vi "Siargo Serial Number.vi"(8 "error in (no error)":errorcluster, 11 "Modbus API in":refnum<class "Modbus API.lvclass">) -> (0 "error out":errorcluster, 2 "Serial Number":string="*G7AEI02058*", 3 "Modbus API out":refnum<class "Modbus API.lvclass">)   [LabVIEW 2020]
uses:
  <vilib>/NI/Modbus Library/API/Modbus API.lvclass
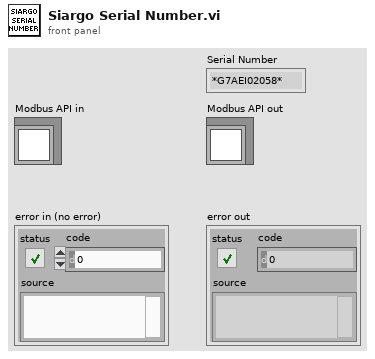
[diagram p1: front panel]
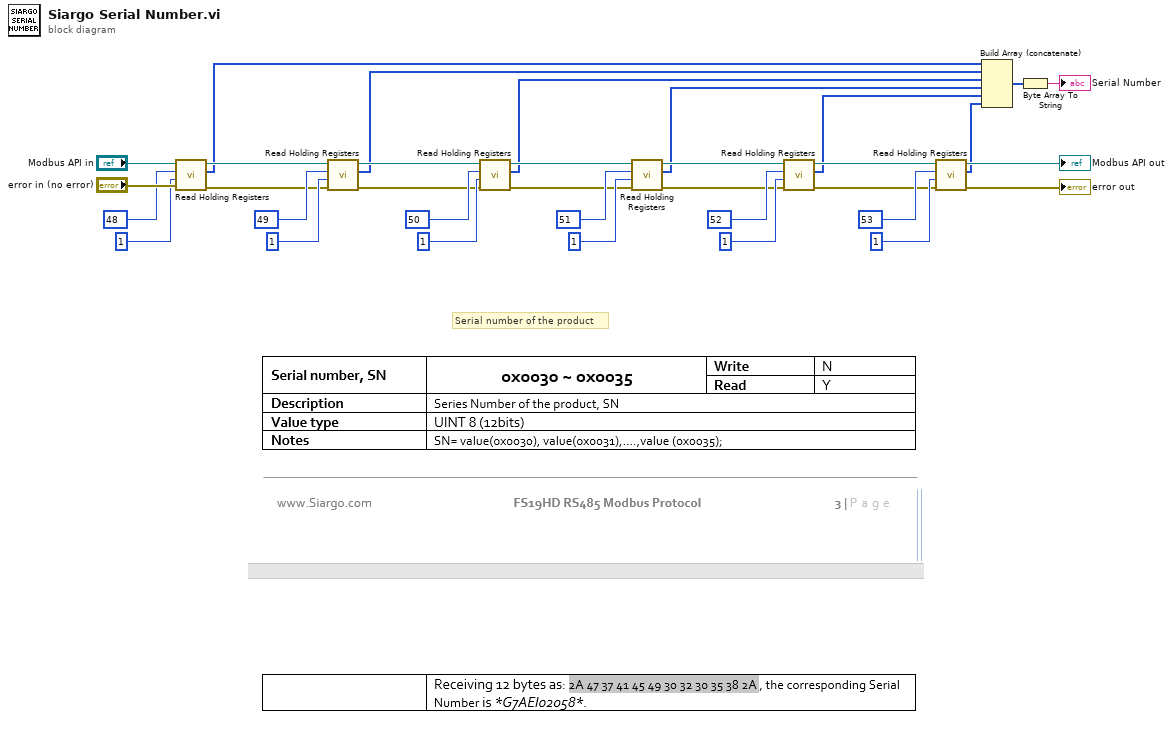
[diagram p0: block diagram]
diagram:
  # "Serial number of the product"
  n1 = call-dynamic "Read Holding Registers.vi"("error in"="error in (no error)", "number of inputs"=u16 1, "starting address"=u16 48, "Modbus instance in"="Modbus API in") -> ("error out"=w20:errorcluster, "register values"=w8:u16[], "Modbus instance out"=w13:refnum<class "Modbus API.lvclass">)  [unwired: 5 in]
  n2 = call-dynamic "Read Holding Registers.vi"("error in"=w20, "number of inputs"=u16 1, "starting address"=u16 49, "Modbus instance in"=w13) -> ("error out"=w19:errorcluster, "register values"=w7:u16[], "Modbus instance out"=w12:refnum<class "Modbus API.lvclass">)  [unwired: 5 in]
  n3 = call-dynamic "Read Holding Registers.vi"("error in"=w19, "number of inputs"=u16 1, "starting address"=u16 50, "Modbus instance in"=w12) -> ("error out"=w18:errorcluster, "register values"=w6:u16[], "Modbus instance out"=w11:refnum<class "Modbus API.lvclass">)  [unwired: 5 in]
  n4 = call-dynamic "Read Holding Registers.vi"("error in"=w18, "number of inputs"=u16 1, "starting address"=u16 51, "Modbus instance in"=w11) -> ("error out"=w17:errorcluster, "register values"=w5:u16[], "Modbus instance out"=w10:refnum<class "Modbus API.lvclass">)  [unwired: 5 in]
  n5 = call-dynamic "Read Holding Registers.vi"("error in"=w17, "number of inputs"=u16 1, "starting address"=u16 52, "Modbus instance in"=w10) -> ("error out"=w16:errorcluster, "register values"=w4:u16[], "Modbus instance out"=w9:refnum<class "Modbus API.lvclass">)  [unwired: 5 in]
  n6 = call-dynamic "Read Holding Registers.vi"("error in"=w16, "number of inputs"=u16 1, "starting address"=u16 53, "Modbus instance in"=w9) -> ("error out"=→"error out":errorcluster, "register values"=w3:u16[], "Modbus instance out"=→"Modbus API out":refnum<class "Modbus API.lvclass">)  [unwired: 5 in]
  n7 = Build Array (concatenate)(w8, w7, w6, w5, w4, w3) -> (w1:u16[])
  n8 = Byte Array To String(unsigned byte array=w1) -> (string=→"Serial Number":string)
